vi "Close Connection.vi"(8 "error in (no error)":errorcluster, 11 "Connection in":refnum<class "Connection.lvclass">) -> (0 "error out":errorcluster, 3 "No Connection":refnum<class "Connection.lvclass">)   [LabVIEW 2013, in "MQTT_Connection.lvlib" / "Connection.lvclass"]
uses:
  Connection.lvclass
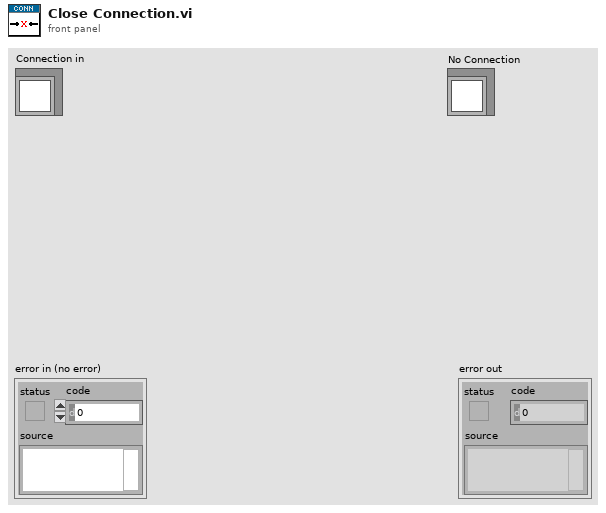
[diagram p1: front panel]
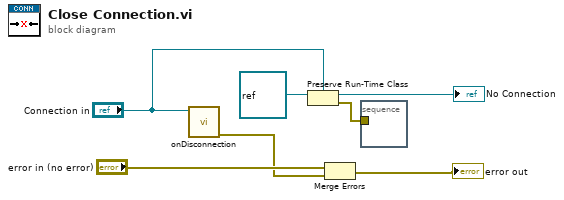
[diagram p0: block diagram]
diagram:
  n1 = call-dynamic "onDisconnection.vi"("Connection"="Connection in") -> ("error out"=w5:errorcluster)  [unwired: 9 in, 1 out]
  n2 = Preserve Run-Time Class(object in=refnum<class> refnum ("LabVIEW Object"), 2:"Connection in") -> (object out=→"No Connection":refnum<class "Connection.lvclass">, error out=w1:errorcluster)  [unwired: 1 in]
  n3 = Merge Errors("error in (no error)", w5) -> (→"error out":errorcluster)
  n4 = stacked-sequence {
    tunnel: w1 -> [_]
    frame #0 {
    }
  }
